vi "TurnForAngle-C.vi"(11 "Params":string[][](array[string])) -> ()   [LabVIEW 2019]
uses:
  Framework/Robot Global Data.vi
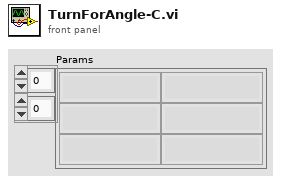
[diagram p1: front panel]
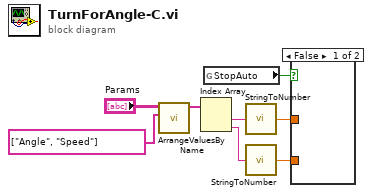
[diagram p0: block diagram]
diagram:
  n1 = call "ArrangeValuesByName.vi"("Names"=string[] ["Angle", "Speed"], "Names/Values in"="Params") -> ("Values Out"=w3:string[])  [unwired: 9 in]
  n2 = Index Array(array=w3) -> (element #1=w2:string, element #2=w1:string)  [unwired: 2 in]
  n3 = global read "Robot Global Data.vi" "StopAuto"() -> (w7:bool)
  n4 = call "StringToNumber.vi"("String"=w2) -> ("Output"=w8:dbl)
  n5 = call "StringToNumber.vi"("String"=w1) -> ("Output"=w6:dbl)
  n6 = case shown="False" w7 {
    tunnel: w8 -> [_ _]
    tunnel: w6 -> [_ _]
    frame False {
    }
    frame True {
    }
  }
